vi "Get VISA Sessions.vi"(8 "Error In":errorcluster) -> (0 "Error Out":errorcluster, 3 "Visa Sources":refnum<visa-resource-name>[](array[refnum]))   [LabVIEW 2014]
uses:
  <vilib>/Instr/_visa.llb/VISA Configure Serial Port (Instr).vi
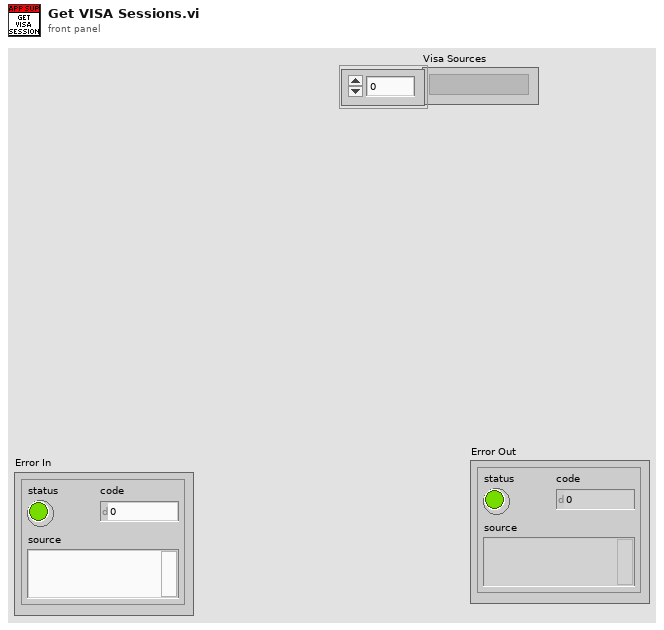
[diagram p1: front panel]
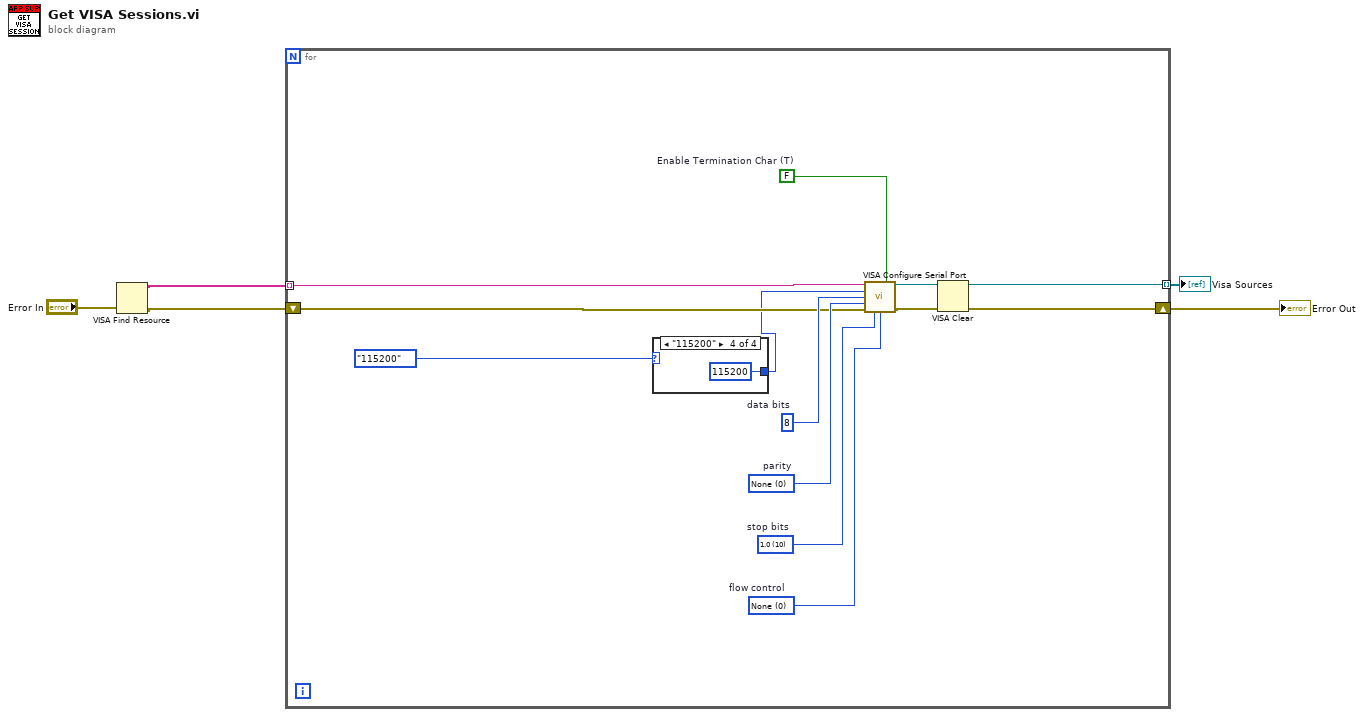
[diagram p0: block diagram]
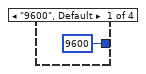
[diagram p2: hidden frame]
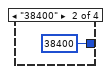
[diagram p3: hidden frame]
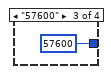
[diagram p4: hidden frame]
diagram:
  n1 = VISA Find Resource(8:"Error In") -> (0:w3:errorcluster, 3:w2:string[])  [unwired: 2 in, 1 out]
  n2 = for {
    shift-right: [w18] -> w5
    shift-left: w3 -> [w9]
    tunnel: [w8] -> w1 mode=indexing
    tunnel: w2 -> [w7] mode=indexing
    w15 = u16 0 items=["None"=0, "XON/XOFF"=1, "RTS/CTS"=2, "DTR/DSR"=4]  # flow control
    w14 = u16 10 items=["1.0"=10, "1.5"=15, "2.0"=20]  # stop bits
    w12 = u16 0 items=["None", "Odd", "Even", "Mark", "Space"]  # parity
    w16 = u16 8  # data bits
    w13 = FALSE  # Enable Termination Char (T)
    n3 = case shown="\"115200\"" enum16{"9600", "38400", "57600", "115200"}."115200" ("Baud Rate") {
      tunnel: [u32 9600 ("baud rate") u32 38400 ("baud rate") u32 57600 ("baud rate") u32 115200 ("baud rate")] -> w6
      frame "9600", Default {
      }
      frame "38400" {
      }
      frame "57600" {
      }
      frame "115200" {
      }
    }
    n4 = call-poly "VISA Configure Serial Port"("VISA resource name"=w7, "Enable Termination\nChar (T)"=w13, "baud rate (9600)"=w6, "data bits (8)"=w16, "parity (0:none)"=w12, "error in (no error)"=w9, "stop bits (10: 1 bit)"=w14, "flow control (0:none)"=w15) -> ("VISA resource name out"=w11:refnum<visa-resource-name>, "error out"=w10:errorcluster)  [unwired: 1 in, 5 out]
    n5 = VISA Clear(VISA resource name=w11, error in (no error)=w10) -> (VISA resource name out=w8:refnum<visa-resource-name>, error out=w18:errorcluster)
  }
  "Error Out" <- w5
  "Visa Sources" <- w1
